vi "2 Garbage Can Auto.vi"(11 "Can Auto Enable":bool) -> ()   [LabVIEW 2014]
uses:
  General_VI/Global Var.vi
panel:
  in  "Time _To_Drive_1_Tote":i32=8000
  in  "Extend_Flipper_Time":i32=500
  in  "Open_Infeed_time":i32=800
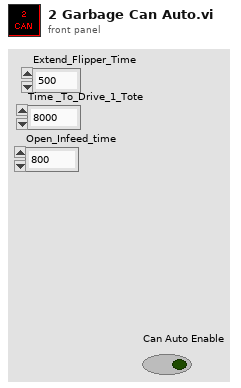
[diagram p1: front panel]
types:
  T1 = cluster{"Open_Infeed_time":i32, "Extend_Flipper_Time":i32, "Time _To_Drive_1_Tote":i32}
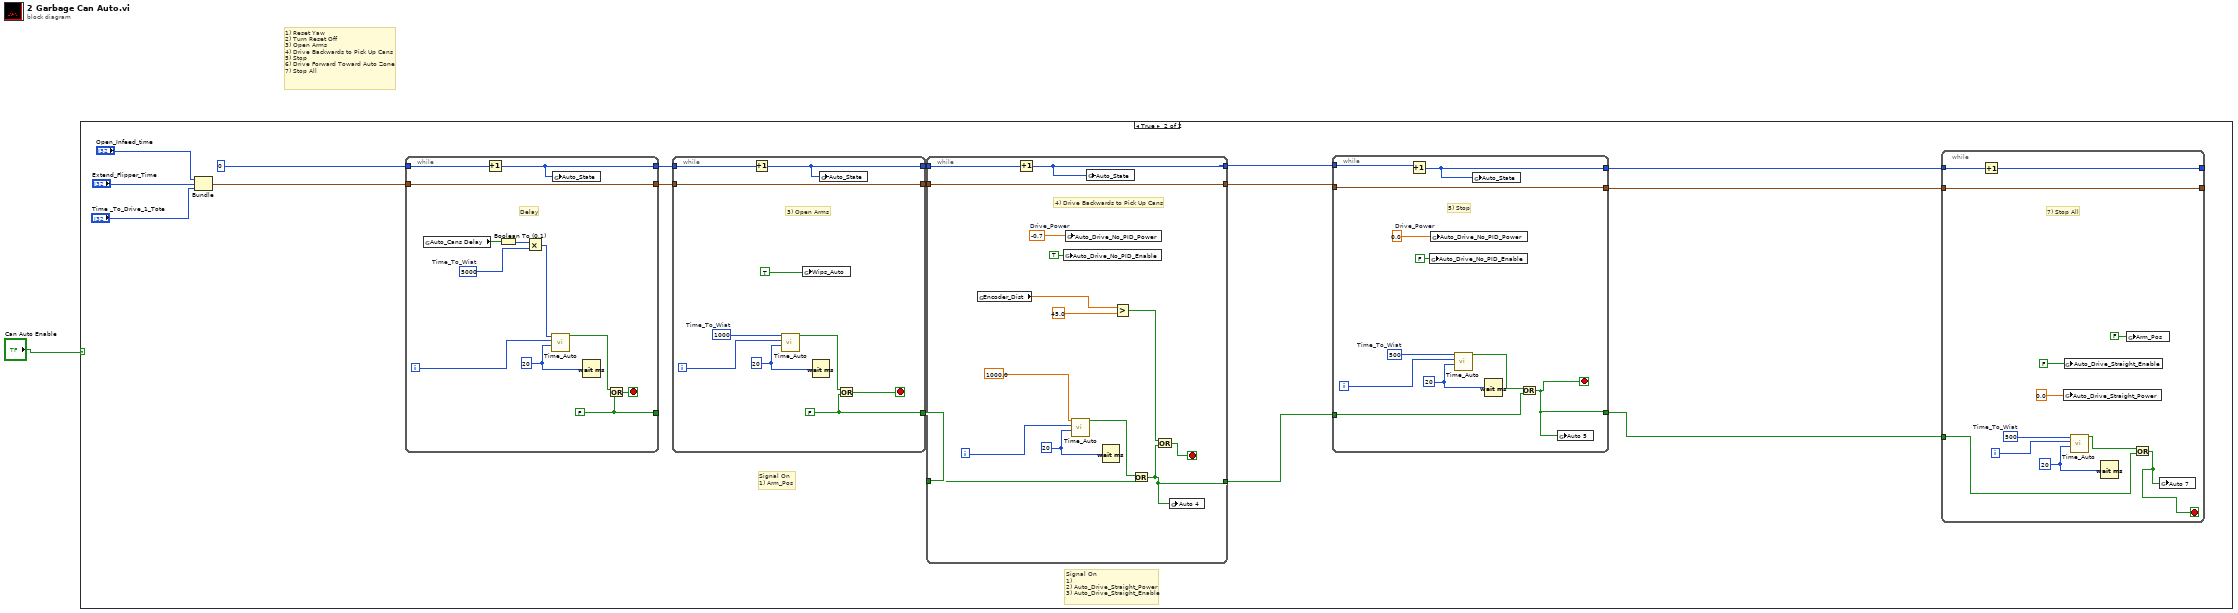
[diagram p0: block diagram]
diagram:
  # "1) Reset Yaw\n2) Turn Reset Off\n3) Open Arms\n4) Drive Backwards to Pick Up Cans\n5) Stop\n6) Drive Forward Toward Auto Zone\n7) Stop All"
  n1 = case shown="True" "Can Auto Enable" {
    frame False {
    }
    frame True {
      # "Signal On\n1) \n2) Auto_Drive_Straight_Power\n3) Auto_Drive_Straight_Enable"
      # "Signal On\n1) Arm_Pos"
      n2 = Bundle("Open_Infeed_time"="Open_Infeed_time", "Extend_Flipper_Time"="Extend_Flipper_Time", "Time _To_Drive_1_Tote"="Time _To_Drive_1_Tote") -> (w2:T1)  [unwired: 1 in]
      n3 = while {
        tunnel: 0 -> [w26]
        tunnel: [w25] -> w5
        tunnel: w2 -> [w27]
        tunnel: [w27] -> w4
        tunnel: [w22] -> _
        i -> [w28]
        stop <- w23 stop-if-true
        w22 = FALSE
        w29 = u32 20 ("milliseconds to wait")
        w19 = 5000  # Time_To_Wiat
        # "Delay"
        n4 = global read "Global Var.vi" "Auto_Cans Delay"() -> (w21:bool)
        n5 = Increment(x=w26) -> (x+1=w25:i32)
        n6 = Boolean To (0,1)(Boolean=w21) -> (0, 1=w20:i16)
        n7 = Multiply(x=w20, y=w19) -> (x*y=w18:i32)
        n8 = call "Time_Auto.vi"("Sample_Time"=w29, "Counter"=w28, "Time_to_wait"=w18) -> ("Boolean"=w24:bool)  [unwired: 8 in]
        n9 = global write "Global Var.vi" "Auto_State"(w25) -> ()
        n10 = Wait (ms)(milliseconds to wait=w29) -> ()  [unwired: 1 out]
        n11 = Or(x=w24, y=w22) -> (x .or. y?=w23:bool)
      }
      n12 = while {
        tunnel: w5 -> [w73]
        tunnel: [w72] -> w14
        tunnel: w4 -> [w74]
        tunnel: [w74] -> w13
        tunnel: [w68] -> w12
        i -> [w76]
        stop <- w69 stop-if-true
        w68 = FALSE
        w77 = u32 20 ("milliseconds to wait")
        w75 = 1000  # Time_To_Wiat
        # "3) Open Arms"
        n13 = Increment(x=w73) -> (x+1=w72:i32)
        n14 = call "Time_Auto.vi"("Sample_Time"=w77, "Counter"=w76, "Time_to_wait"=w75) -> ("Boolean"=w71:bool)  [unwired: 8 in]
        n15 = global write "Global Var.vi" "Wips_Auto"(TRUE) -> ()
        n16 = Wait (ms)(milliseconds to wait=w77) -> ()  [unwired: 1 out]
        n17 = global write "Global Var.vi" "Auto_State"(w72) -> ()
        n18 = Or(x=w71, y=w68) -> (x .or. y?=w69:bool)
      }
      n19 = while {
        tunnel: [w59] -> w11
        tunnel: w14 -> [w60]
        tunnel: [w67] -> w10
        tunnel: w13 -> [w67]
        tunnel: w12 -> [w64]
        tunnel: [w61] -> w9
        i -> [w65]
        stop <- w62 stop-if-true
        w53 = -0.7  # Drive_Power
        w66 = u32 20 ("milliseconds to wait")
        # "4) Drive Backwards to Pick Up Cans"
        n20 = global read "Global Var.vi" "Encoder_Dist"() -> (w58:dbl)
        n21 = Increment(x=w60) -> (x+1=w59:i32)
        n22 = global write "Global Var.vi" "Auto_Drive_No_PID_Enable"(TRUE ("Auto_Drive_No_PID_Enable")) -> ()
        n23 = global write "Global Var.vi" "Auto_Drive_No_PID_Power"(w53) -> ()
        n24 = call "Time_Auto.vi"("Sample_Time"=w66, "Counter"=w65, "Time_to_wait"=1000.0) -> ("Boolean"=w63:bool)  [unwired: 8 in]
        n25 = global write "Global Var.vi" "Auto_State"(w59) -> ()
        n26 = Wait (ms)(milliseconds to wait=w66) -> ()  [unwired: 1 out]
        n27 = Greater?(x=w58, y=45.0) -> (0:w56:bool)
        n28 = Or(x=w63, y=w64) -> (x .or. y?=w61:bool)
        n29 = Or(x=w56, y=w61) -> (x .or. y?=w62:bool)
        n30 = global write "Global Var.vi" "Auto 4"(w61) -> ()
      }
      n31 = while {
        tunnel: w11 -> [w47]
        tunnel: [w52] -> w7
        tunnel: w10 -> [w52]
        tunnel: w9 -> [w45]
        tunnel: [w46] -> w8
        tunnel: [w44] -> w6
        i -> [w49]
        stop <- w44 stop-if-true
        w42 = 0.0  # Drive_Power
        w51 = u32 20 ("milliseconds to wait")
        w50 = 500  # Time_To_Wiat
        # "5) Stop"
        n32 = Increment(x=w47) -> (x+1=w46:i32)
        n33 = global write "Global Var.vi" "Auto_Drive_No_PID_Enable"(FALSE ("Auto_Drive_No_PID_Enable")) -> ()
        n34 = global write "Global Var.vi" "Auto_Drive_No_PID_Power"(w42) -> ()
        n35 = call "Time_Auto.vi"("Sample_Time"=w51, "Counter"=w49, "Time_to_wait"=w50) -> ("Boolean"=w48:bool)  [unwired: 8 in]
        n36 = global write "Global Var.vi" "Auto_State"(w46) -> ()
        n37 = Wait (ms)(milliseconds to wait=w51) -> ()  [unwired: 1 out]
        n38 = Or(x=w48, y=w45) -> (x .or. y?=w44:bool)
        n39 = global write "Global Var.vi" "Auto 5"(w44) -> ()
      }
      n40 = while {
        tunnel: w8 -> [w41]
        tunnel: [w40] -> _
        tunnel: [w39] -> _
        tunnel: w7 -> [w39]
        tunnel: w6 -> [w31]
        i -> [w36]
        stop <- w30 stop-if-true
        w38 = u32 20 ("milliseconds to wait")
        w37 = 500  # Time_To_Wiat
        # "7) Stop All"
        n41 = Increment(x=w41) -> (x+1=w40:i32)
        n42 = global write "Global Var.vi" "Auto_Drive_Straight_Power"(0.0 ("Auto_Drive_Straight_Power")) -> ()
        n43 = global write "Global Var.vi" "Auto_Drive_Straight_Enable"(FALSE ("Auto_Drive_Straight_Enable")) -> ()
        n44 = call "Time_Auto.vi"("Sample_Time"=w38, "Counter"=w36, "Time_to_wait"=w37) -> ("Boolean"=w32:bool)  [unwired: 8 in]
        n45 = Wait (ms)(milliseconds to wait=w38) -> ()  [unwired: 1 out]
        n46 = global write "Global Var.vi" "Arm_Pos"(FALSE ("Arm_Pos")) -> ()
        n47 = Or(x=w32, y=w31) -> (x .or. y?=w30:bool)
        n48 = global write "Global Var.vi" "Auto 7"(w30) -> ()
      }
    }
  }
